vi "Shooter Control wPID Ryan Green Version.vi"() -> ()   [LabVIEW 2016]
uses:
  Robot Values.vi
  <vilib>/addons/control/pid/pid.llb/PID (DBL).vi
  <vilib>/addons/control/pid/NI_PID_pid.lvlib
  <vilib>/ptbypt/NI_PtbyPt.lvlib
panel:
  in  "Agitate State":enum16{"In", "Out"}(ring)
  in  "Agitate Out SP":dbl=-0.5
  in  "Agitate In SP":dbl=0.5
  in  "Aquisition Power":dbl=0.7
  in  "Baseline Power":dbl=0.48 format="%#_13g"
  in  "Time Target (s)":dbl=0.15 format="%#_13g"
  in  "PID gains":T1={"proportional gain (Kc)"=1.0, "integral time (Ti, min)"=0.01, "derivative time (Td, min)"=0.0} {"derivative time (Td, min)" format="%.3f"; "integral time (Ti, min)" format="%.3f"; "proportional gain (Kc)" format="%.3f"}
  in  "setpoint":dbl format="%#_13g"
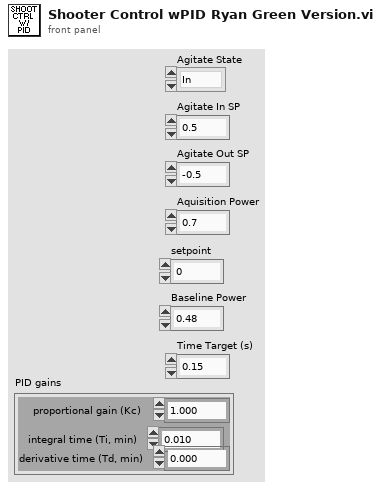
[diagram p1: front panel]
types:
  T1 = cluster{"proportional gain (Kc)":dbl, "integral time (Ti, min)":dbl, "derivative time (Td, min)":dbl}
  T2 = typedef "Robot Values.ctl" = cluster{"Robot Drive":cluster{"Left Motor Power":dbl, "Right Motor Power":dbl, "Left Encoder Value":dbl, "Right Encoder Value":dbl, "High Gear?":bool, "PTO?":bool}, "Sensors":cluster{"Gyro Angle":dbl, "Recalibrate Gyro":bool, "Reset Gyro":bool}, "Shooter":cluster{"Prep Wheels":bool, "Shoot":bool, "Left Shooter Wheel Speed":dbl, "Right Shooter Wheel Speed":dbl, "Wheels Moving":bool, "Shooter Prepped":bool, "Shooter RPS SP":dbl, "Aquiring?":bool, "Shooting?":bool, "Left Shooter Wheel Power":dbl, "Right Shooter Wheel Power":dbl, "Acquisition Conveyor Power":dbl, "Hopper Beater Bar Power":dbl}, "Robot States":cluster{"Drive mode":string, "Alliance":T3, "Position":T4}, "Gear":cluster{"Ejection Active":bool}, "Lights":cluster{"Current Light State":string}}
  T3 = typedef "WPI_DriverStationAllianceInfo.ctl" = enum16{"Red", "Blue", "Invalid"}
  T4 = typedef "WPI_DriverStationPositionInfo.ctl" = enum16{"1", "2", "3"}
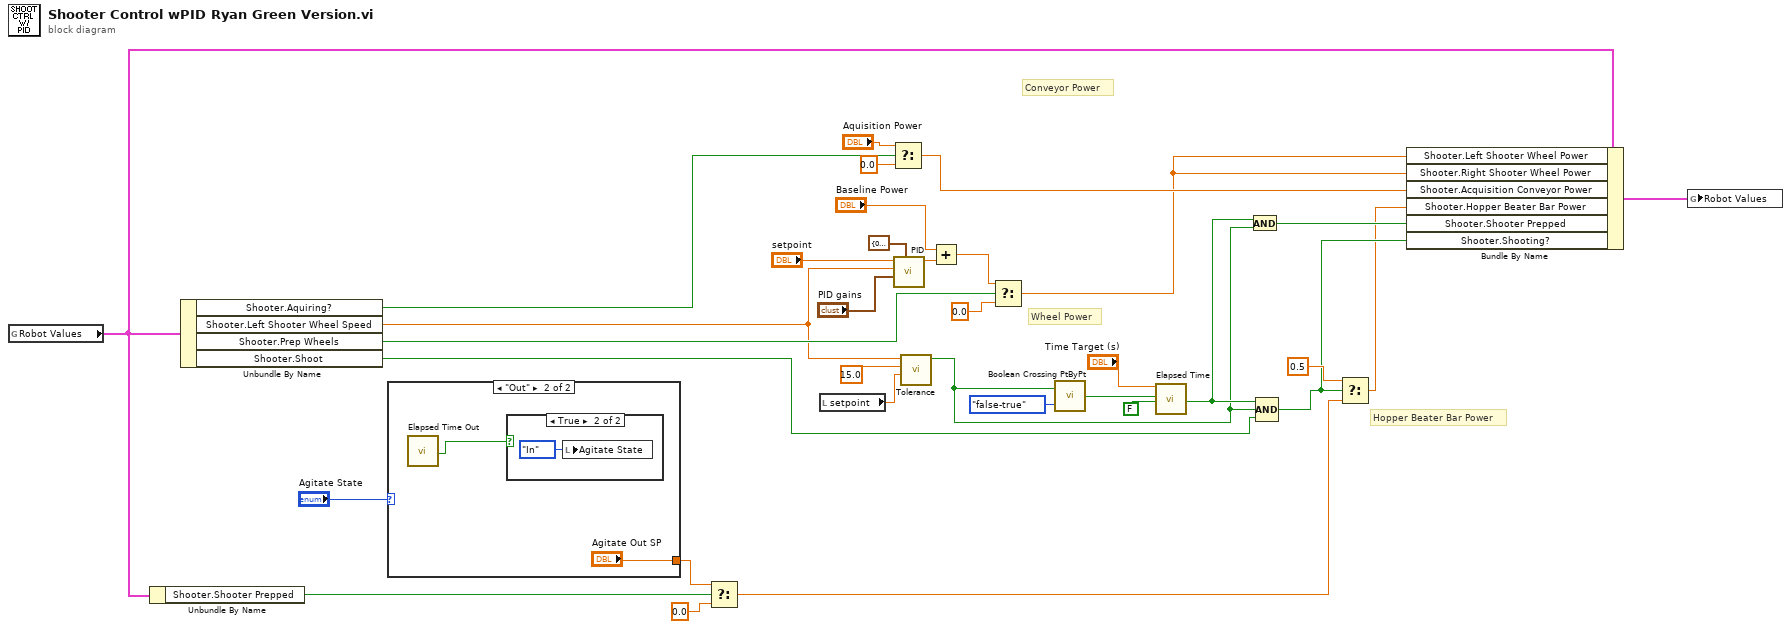
[diagram p0: block diagram]
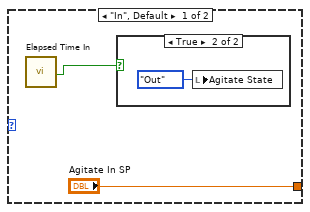
[diagram p2: hidden frame]
diagram:
  # "Hopper Beater Bar Power"
  # "Conveyor Power"
  # "Wheel Power"
  n1 = global read "Robot Values.vi" "Robot Values"() -> (w10:T2)
  n2 = Unbundle By Name(w10) -> ("Shooter.Shooter Prepped"=w6:bool)
  n3 = Unbundle By Name(w10) -> ("Shooter.Aquiring?"=w13:bool, "Shooter.Left Shooter Wheel Speed"=w21:dbl, "Shooter.Prep Wheels"=w34:bool, "Shooter.Shoot"=w19:bool)
  n4 = case shown="\"Out\"" "Agitate State" {
    tunnel: ["Agitate In SP" "Agitate Out SP"] -> w3
    frame "In", Default {
      n5 = call "Elapsed Time In"() -> ("Time has Elapsed"=w35:bool)  [unwired: 12 in, 7 out]
      n6 = case shown="True" w35 {
        frame False {
        }
        frame True {
          n7 = local write "Agitate State"(enum16{"In", "Out"}."Out" ("Agitate State")) -> ()
        }
      }
    }
    frame "Out" {
      n8 = call "Elapsed Time Out"() -> ("Time has Elapsed"=w38:bool)  [unwired: 12 in, 7 out]
      n9 = case shown="True" w38 {
        frame False {
        }
        frame True {
          n10 = local write "Agitate State"(enum16{"In", "Out"}."In" ("Agitate State")) -> ()
        }
      }
    }
  }
  n11 = Select(t=w3, s=w6, f=0.0) -> (s? t:f=w1:dbl)
  n12 = local read "setpoint"() -> (w20:dbl)
  n13 = Select(t="Aquisition Power", s=w13, f=0.0) -> (s? t:f=w8:dbl)
  n14 = call-poly <vilib>:"PID.vi"("output range"=cluster{"output high":dbl, "output low":dbl} {"output high"=0.1, "output low"=-0.1}, "PID gains"="PID gains", "process variable"=w21, "setpoint"="setpoint") -> ("output"=w31:dbl)  [unwired: 6 in, 1 out]
  n15 = call "Tolerance.vi"("Setpoint"=w20, "Tolerance"=15.0, "Current Value"=w21) -> ("In Range?"=w16:bool)  [unwired: 8 in]
  n16 = Add(x="Baseline Power", y=w31) -> (x+y=w32:dbl)
  n17 = Select(t=w32, s=w34, f=0.0) -> (s? t:f=w7:dbl)
  n18 = call <vilib>:"Boolean Crossing PtByPt.vi"("direction"=enum16{"either", "false-true", "true-false"}."false-true", "input"=w16) -> ("crossing"=w24:bool)  [unwired: 1 in]
  n19 = call "Elapsed Time"("Time Target (s)"="Time Target (s)", "Reset"=w24, "Auto Reset"=FALSE) -> ("Time has Elapsed"=w17:bool)  [unwired: 9 in, 7 out]
  n20 = And(x=w17, y=w16) -> (x .and. y?=w15:bool)
  n21 = Compound Arithmetic op=AND(w17, w16, w19) -> (w11:bool)
  n22 = Select(t=0.5, s=w11, f=w1) -> (s? t:f=w9:dbl)
  n23 = Bundle By Name(cluster=w10, "Shooter.Left Shooter Wheel Power"=w7, "Shooter.Right Shooter Wheel Power"=w7, "Shooter.Acquisition Conveyor Power"=w8, "Shooter.Hopper Beater Bar Power"=w9, "Shooter.Shooter Prepped"=w15, "Shooter.Shooting?"=w11) -> (w14:T2)
  n24 = global write "Robot Values.vi" "Robot Values"(w14) -> ()
